vi "pattern_hcp_shack_hartmann.vi"(6 "Width":dbl=3e-05, 9 "Reference Array?":bool, 10 "Fraction of SLM":dbl=1.0, 11 "N":i32=5) -> (3 "Shack-Hartmann Spots":T1[](array[typedef]) {"Amplitude Correction" step=0.1; "Line Trapping"."Phase Gradient" step=0.05; "Line Trapping"."Vector"."x" step=1e-06 format="%#_6p"; "Line Trapping"."Vector"."y" step=1e-06 format="%#_6p"; "Line Trapping"."Vector"."z" step=1e-06 format="%#_6p"; "NA Position"."r" step=1e-06; "NA Position"."y" step=1e-06; "NA Position"."x" step=1e-06; "Position"."z" step=1e-06; "Position"."y" step=1e-06; "Position"."x" step=1e-06; "Phase" step=0.7753; "Intensity" step=0.1})   [LabVIEW 2010]
uses:
  spot.ctl
  line_trapping.ctl
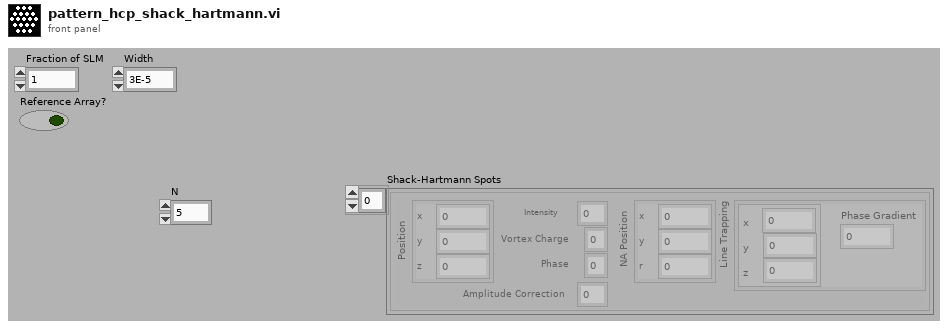
[diagram p1: front panel]
types:
  T1 = typedef "spot.ctl" = cluster{"Position":cluster{"x":dbl, "y":dbl, "z":dbl}, "Intensity":dbl, "Vortex Charge":i8, "Phase":dbl, "NA Position":cluster{"x":dbl, "y":dbl, "r":dbl}, "Line Trapping":T2, "Amplitude Correction":dbl}
  T2 = typedef "line_trapping.ctl" = cluster{"Vector":cluster{"x":dbl, "y":dbl, "z":dbl}, "Phase Gradient":dbl}
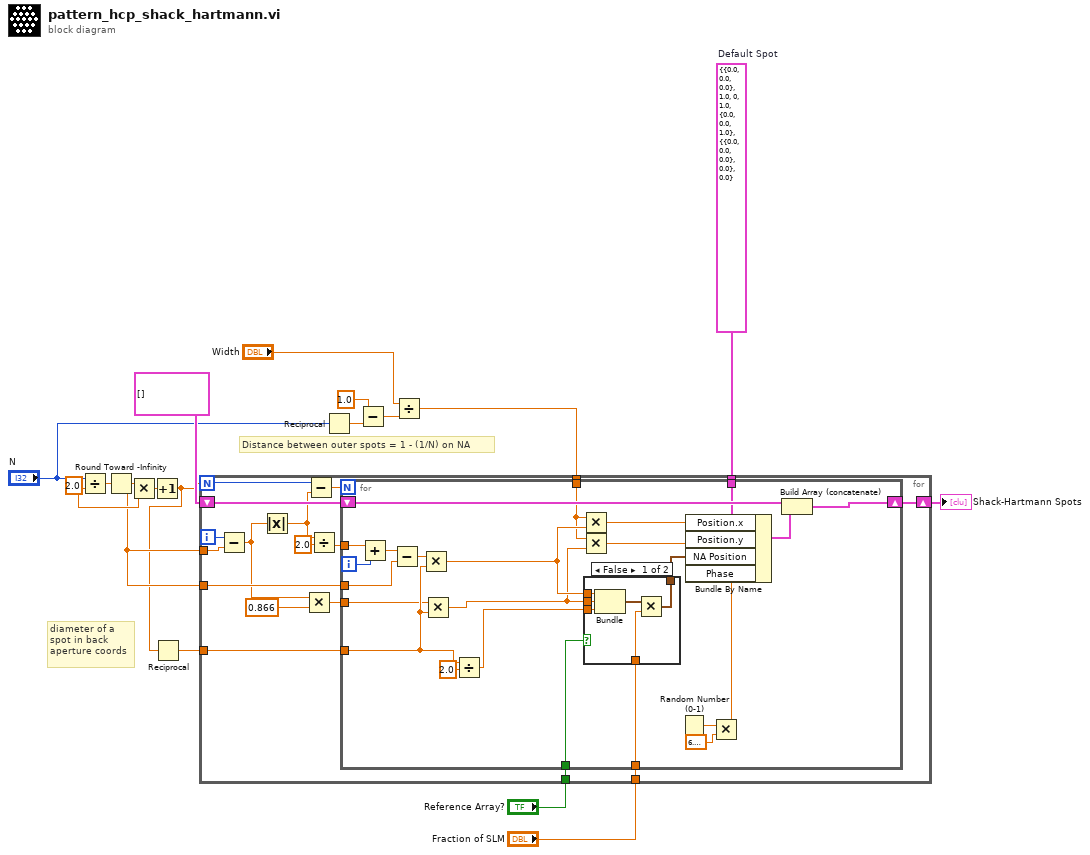
[diagram p0: block diagram]
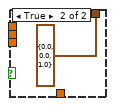
[diagram p2: hidden frame]
diagram:
  w12 = 2.0 ("x")
  w16 = T1 {"Position"={"x"=0.0, "y"=0.0, "z"=0.0}, "Intensity"=1.0, "Vortex Charge"=0, "Phase"=1.0, "NA Position"={"x"=0.0, "y"=0.0, "r"=1.0}, "Line Trapping"={"Vector"={"x"=0.0, "y"=0.0, "z"=0.0}, "Phase Gradient"=0.0}, "Amplitude Correction"=0.0}  # Default Spot
  # "Distance between outer spots = 1 - (1/N) on NA"
  # "diameter of a\nspot in back \naperture coords"
  n1 = Divide(x="N", y=w12) -> (x/y=w15:dbl)
  n2 = Round Toward -Infinity(1:w15) -> (0:w11:dbl)
  n3 = Multiply(x=w11, y=w12) -> (x*y=w14:dbl)
  n4 = Increment(x=w14) -> (x+1=w10:dbl)
  n5 = Reciprocal(x=w10) -> (1/x=w13:dbl)
  n6 = Reciprocal(x="N") -> (1/x=w6:dbl)
  n7 = Subtract(x=1.0, y=w6) -> (x-y=w3:dbl)
  n8 = Divide(x="Width", y=w3) -> (x/y=w1:dbl)
  n9 = for {
    N: w10 -> [w28]
    shift-right: [w34] -> w9
    shift-left: T1[] [] ("Spots") -> [w35]
    tunnel: w16 -> [w33]
    tunnel: w13 -> [w32]
    tunnel: w11 -> [w30]
    tunnel: w11 -> [w24]
    tunnel: "Fraction of SLM" -> [w20]
    tunnel: "Reference Array?" -> [w19]
    tunnel: w1 -> [w18]
    i -> [w31]
    n10 = Subtract(x=w31, y=w30) -> (x-y=w21:dbl)
    n11 = Absolute Value(x=w21) -> (abs(x)=w26:dbl)
    n12 = Multiply(x=w21, y=0.866) -> (x*y=w23:dbl)
    n13 = Subtract(x=w28, y=w26) -> (x-y=w29:dbl)
    n14 = Divide(x=w26, y=2.0 ("x")) -> (x/y=w25:dbl)
    n15 = for {
      N: w29 -> [_]
      shift-right: [w59] -> w34
      shift-left: w35 -> [w58]
      tunnel: w33 -> [w56]
      tunnel: w32 -> [w45]
      tunnel: w25 -> [w49]
      tunnel: w24 -> [w47]
      tunnel: w23 -> [w44]
      tunnel: w20 -> [w38]
      tunnel: w19 -> [w37]
      tunnel: w18 -> [w36]
      i -> [w50]
      n16 = Add(x=w49, y=w50) -> (x+y=w48:dbl)
      n17 = Subtract(x=w48, y=w47) -> (x-y=w46:dbl)
      n18 = Multiply(x=w46, y=w45) -> (x*y=w43:dbl)
      n19 = Multiply(x=w44, y=w45) -> (x*y=w42:dbl)
      n20 = Divide(x=w45, y=2.0 ("x")) -> (x/y=w41:dbl)
      n21 = Multiply(x=w36, y=w43) -> (x*y=w55:dbl)
      n22 = Multiply(x=w36, y=w42) -> (x*y=w54:dbl)
      n23 = case shown="False" w37 {
        tunnel: w43 -> [w65 _]
        tunnel: w42 -> [w64 _]
        tunnel: w41 -> [w63 _]
        tunnel: [w62 cluster{dbl, dbl, dbl} {0.0, 0.0, 1.0} ("output cluster")] -> w39
        tunnel: w38 -> [w60 _]
        frame False {
          n24 = Bundle(w65, w64, w63) -> (w61:cluster{dbl, dbl, dbl})  [unwired: 1 in]
          n25 = Multiply(x=w61, y=w60) -> (x*y=w62:cluster{dbl, dbl, dbl})
        }
        frame True {
        }
      }
      n26 = Random Number (0-1)() -> (number: 0 to 1=w53:dbl)
      n27 = Multiply(x=w53, y=6.283185307179586) -> (x*y=w40:dbl)
      n28 = Bundle By Name(cluster=w56, "Position.x"=w55, "Position.y"=w54, "NA Position"=w39, "Phase"=w40) -> (w57:T1)
      n29 = Build Array (concatenate)(w58, w57) -> (w59:T1[])
    }
  }
  "Shack-Hartmann Spots" <- w9
